vi "Disconnect.vi"(8 "error in (no error)":errorcluster, 11 "VideoScanCamera in":refnum<class "VideoScanDeviceLibrary.lvclass">) -> (0 "error out":errorcluster, 3 "VideoScanCamera out":refnum<class "VideoScanDeviceLibrary.lvclass">)   [LabVIEW 2014, in "VideoScanDeviceLibrary.lvclass"]
uses:
  VideoScanDeviceLibrary.lvclass
  VideoScanDeviceLibrary.lvclass/VideoScanDeviceLibrary.ctl
  <vilib>/MediaMongrels Ltd/WebSockets/WebSockets/WebSockets.lvlib
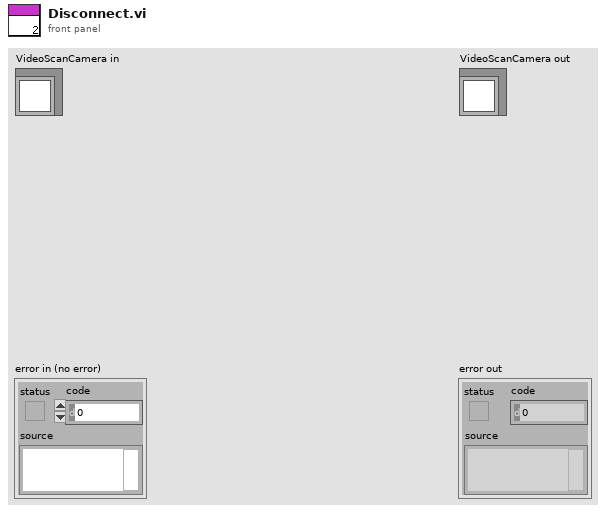
[diagram p1: front panel]
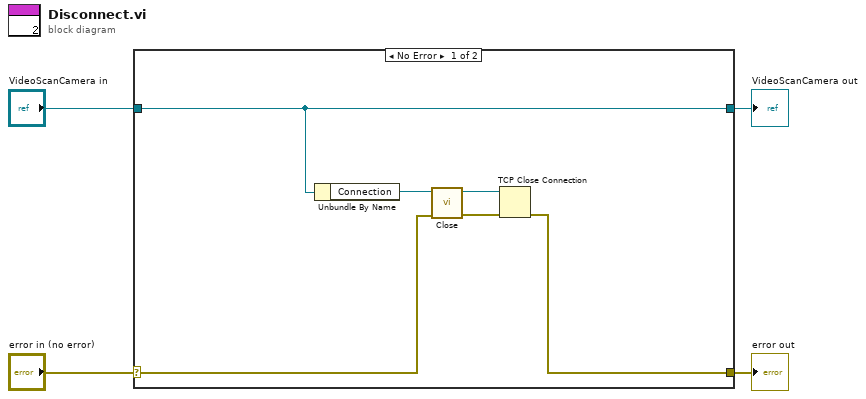
[diagram p0: block diagram]
diagram:
  n1 = case shown="No Error" "error in (no error)" {
    selector: "error in (no error)" -> [w8 w12]
    tunnel: [w7 w12] -> w3
    tunnel: [w5 w11] -> w1
    tunnel: "VideoScanCamera in" -> [w5 w11]
    frame No Error {
      n2 = Unbundle By Name(w5) -> ("Connection"=w6:refnum<k5>)
      n3 = call <vilib>:"Close.vi"("error in (no error)"=w8, "WebSocket Connection in"=w6) -> ("error out"=w9:errorcluster, "WebSocket Connection in"=w10:refnum<k5>)  [unwired: 8 in]
      n4 = TCP Close Connection(connection ID=w10, error in (no error)=w9) -> (error out=w7:errorcluster)  [unwired: 1 in, 1 out]
    }
    frame Error {
    }
  }
  "error out" <- w3
  "VideoScanCamera out" <- w1
